vi "Global 1.vi"() -> ()   [LabVIEW 2021]
panel:
  out "VISA resource name":refnum<visa-resource-name>
  out "Display":string
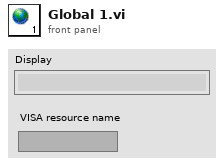
[diagram p1: front panel]
diagram:
